vi "LVClass_Image get image data Uxx.vi"(0 "Image in":refnum<class "Image.lvclass">, 11 "error in (no error)":errorcluster) -> (4 "Image out":refnum<class "Image.lvclass">, 6 "Image data out":u32[][](array[numeric]), 15 "error out":errorcluster)   [LabVIEW 2020, in "Image.lvclass"]
doc: "Get pixels buffer from 32-bit Image.\n\n--------------------------------------------------------------------------------\n\n<B>ImageIn </B> : Image object.\n<B>ImageOut </B> : Image object.\n<B>buffer </B> : Pixel buffer.\n<B>ErrorIn </B> : Error\n<B>ErrorOut </B> : Error\n\n--------------------------------------------------------------------------------"
uses:
  Image.lvclass
  Point2D.ctl
  Image.lvclass/Image.ctl
  LVClass_Image Read Image.vi
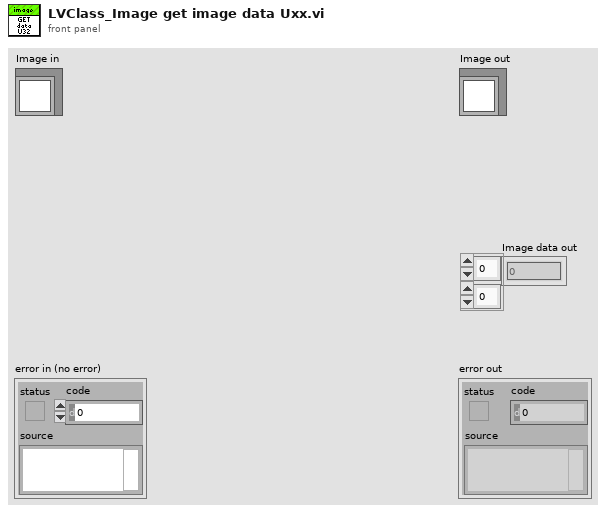
[diagram p1: front panel]
types:
  T1 = typedef "Point2D.ctl" = cluster{"X":u32, "Y":u32}
  T2 = typedef "Struct_Image.ctl" = cluster{"Image_Handler":T3, "Number of bits":T4, "ImageSize":T1}
  T3 = typedef "ClassID.ctl" = i64
  T4 = typedef "Data alignment enum.ctl" = enum16{"8", "16", "32"}
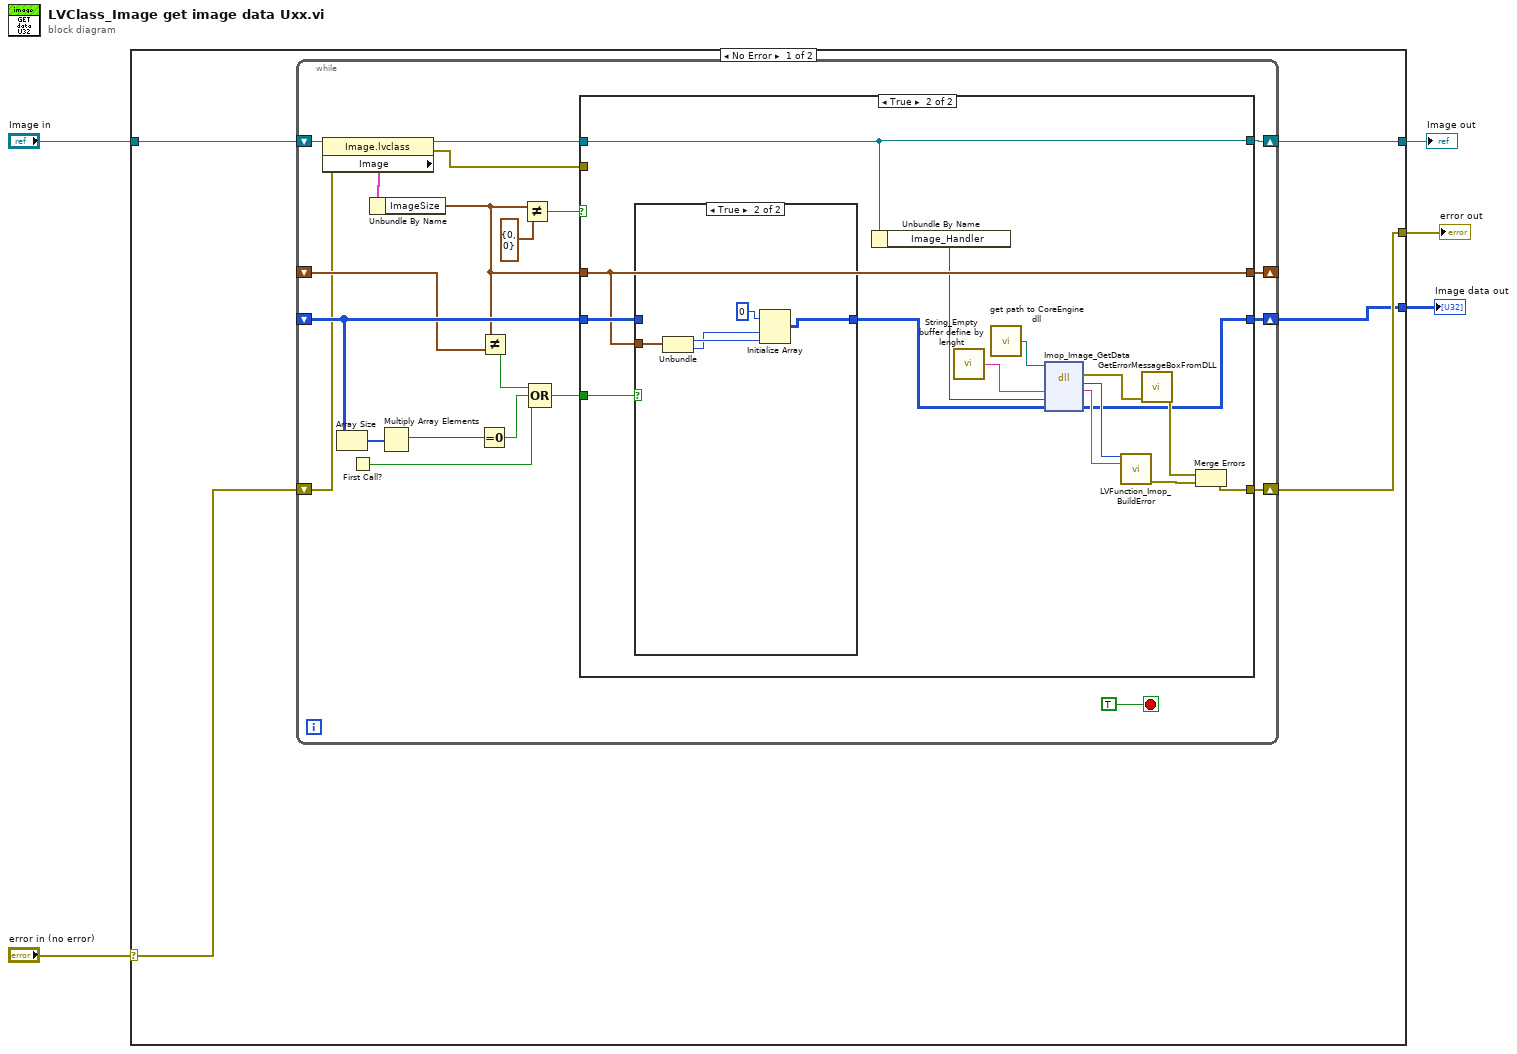
[diagram p0: block diagram]
diagram:
  n1 = case shown="No Error" "error in (no error)" {
    selector: "error in (no error)" -> [w6 w58]
    tunnel: [w9 w58] -> w4
    tunnel: [w8 w57] -> w2
    tunnel: "Image in" -> [w10 w57]
    tunnel: [w7 _] -> w1
    frame No Error {
      n2 = while {
        shift-right: [w31] -> w7
        shift-left: _ -> [w29]
        shift-right: [w23] -> w8
        shift-left: w10 -> [w19]
        shift-right: [w22] -> w9
        shift-left: w6 -> [w18]
        shift-right: [w15] -> _
        shift-left: _ -> [w21]
        stop <- TRUE stop-if-true
        n3 = property class="Image.lvclass"(reference=w19, error in=w18) -> (reference out=w20:refnum<class "Image.lvclass">, error out=w13:errorcluster, "Image"=w14:T2)
        n4 = Array Size(array=w29) -> (size(s)=w28:i32[])
        n5 = First Call?() -> (First Call?: T/F=w25:bool)
        n6 = Unbundle By Name(w14) -> ("ImageSize"=w12:T1)
        n7 = Multiply Array Elements(1:w28) -> (0:w27:i32)
        n8 = Equal To 0?(x=w27) -> (x = 0?=w26:bool)
        n9 = Not Equal?(x=w12, y=w21) -> (x != y?=w11:bool)
        n10 = Not Equal?(x=w12, y=T1 {"X"=0, "Y"=0}) -> (x != y?=w16:bool)
        n11 = Compound Arithmetic op=OR(w11, w26, w25) -> (w24:bool)
        n12 = case shown="True" w16 {
          tunnel: [w35 w36] -> w31
          tunnel: w29 -> [w35 w50]
          tunnel: w24 -> [_ w49]
          tunnel: [w34 w48] -> w23
          tunnel: [w33 w47] -> w22
          tunnel: w20 -> [w34 w48]
          tunnel: w13 -> [w33 _]
          tunnel: w12 -> [w32 w46]
          tunnel: [w32 w46] -> w15
          frame False {
          }
          frame True {
            n13 = case shown="True" w49 {
              tunnel: [w51 w56] -> w37
              tunnel: w50 -> [w51 _]
              tunnel: w46 -> [_ w55]
              frame False {
              }
              frame True {
                n14 = Unbundle(w55) -> ("X"=w54:u32, "Y"=w53:u32)
                n15 = Initialize Array(u32 0 ("element"), w53, w54) -> (w56:u32[][])
              }
            }
            n16 = Unbundle By Name(w48) -> ("Image_Handler"=w45:T3)
            n17 = call "String_Empty buffer define by lenght.vi"() -> ("Empty buffer"=w38:string)  [unwired: 1 in]
            n18 = call "get path to CoreEngine dll.vi"() -> ("path to wavekit library"=w39:path)  [unwired: 14 in, 1 out]
            n19 = dll-call lib="D:/soft/HASO_v3/SVN_trunk/ImOpCoreEngine4_LV2011/DLLs/c_interface_vc100.dll" fn="Imop_Image_GetData"(path in=w39, "message"=w38, "Image compat"=w45, "Image data"=w37) -> (error out=w40:errorcluster, "return type"=w42:i32, "message"=w41:string, "Image data"=w36:u32[][])  [unwired: 3 in, 1 out]
            n20 = call "LVFunction_Imop_BuildError.vi"("code"=w42, "String to Prepend to source (\"\")"=w41) -> ("error out"=w44:errorcluster)  [unwired: 13 in]
            n21 = call "GetErrorMessageBoxFromDLL.vi"("error IN"=w40) -> ("error OUT"=w43:errorcluster)  [unwired: 10 in]
            n22 = Merge Errors(w43, w44) -> (w47:errorcluster)
          }
        }
      }
    }
    frame Error {
    }
  }
  "error out" <- w4
  "Image out" <- w2
  "Image data out" <- w1
